vi "get results seq channel list.vi"(11 "engine configuration in":refnum<class "base TBM sequencer configuration.lvclass">) -> (2 "restults seq channels":refnum<class "TBM channel.lvclass">[](array[class]), 3 "engine configuration out":refnum<class "base TBM sequencer configuration.lvclass">)   [LabVIEW 2014, in "base TBM sequencer configuration.lvclass"]
uses:
  base TBM sequencer configuration.lvclass
  <vilib>/NI/Tag Bus Module Framework/channel/TBM channel.lvclass
  base TBM sequencer configuration.lvclass/base TBM sequencer configuration.ctl
  <vilib>/NI/Tag Bus Module Framework/channel/channel classification.ctl
  <vilib>/NI/Tag Bus Module Framework/channel/TBM channel.lvclass/TBM channel.ctl
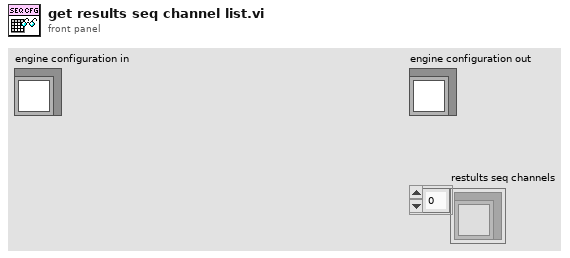
[diagram p1: front panel]
types:
  T1 = typedef "base TBM sequencer configuration.lvclass/Tag Info.ctl" = cluster{"Channel":refnum<class "TBM channel.lvclass">, "Writers":string[], "Readers":string[], "Owning ID":string}
  T2 = typedef "TBM channel.lvclass/channel classification.ctl" = enum16{"input data", "output data", "processing parameter", "processing result"}
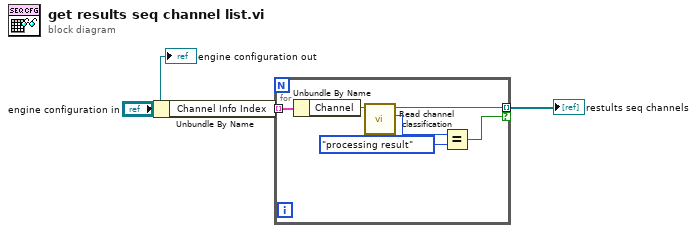
[diagram p0: block diagram]
diagram:
  n1 = Unbundle By Name("engine configuration in") -> ("Channel Info Index"=w3:T1[])
  n2 = for {
    tunnel: w3 -> [w9] mode=indexing
    tunnel: [w7] -> w2 mode=indexing if=w4
    n3 = Unbundle By Name(w9) -> ("Channel"=w8:refnum<class "TBM channel.lvclass">)
    n4 = call <vilib>:"Read channel classification.vi"("channel in"=w8) -> ("channel classification"=w6:T2, "channel out"=w7:refnum<class "TBM channel.lvclass">)  [unwired: 8 in, 1 out]
    n5 = Equal?(x=w6, y=channel_classification."processing result") -> (x = y?=w4:bool)
  }
  "restults seq channels" <- w2
  "engine configuration out" <- "engine configuration in"
